vi "Begin.vi"(8 "error in":errorcluster) -> (0 "error out":errorcluster)   [LabVIEW 2014]
doc: "Called before other user functions, this VI is expected to open initial I/O refnums, load in file data, and do all program initialization. Notice that the <B>error out</B> terminal is simply used for data flow. Wiring it to other structures or subVIs ensures that this VI runs first."
uses:
  <vilib>/Rock Robotics/WPI/DriverStation/WPI_DriverStationRobotMode2.ctl
  <vilib>/Rock Robotics/WPI/Joystick/WPI_JoystickDeviceEnum.ctl
  <vilib>/Rock Robotics/WPI/CAN/TalonSRX/WPI_CANTalonSRX_APIControlMode.ctl
  <vilib>/Rock Robotics/WPI/RobotDrive/WPI_RobotDriveMotorSelectorEnum.ctl
  <vilib>/Rock Robotics/SystemInterfaces/Typedef/FPGA_TypedefDigitalModule.ctl
  Robot Global Data.vi
  <vilib>/Rock Robotics/WPI/Compressor/WPI_CompressorGetSetRefNum.vi
  <vilib>/Rock Robotics/WPI/MotorControl/WPI_MotorControlOpenCANTalonSRX.vi
  <vilib>/Rock Robotics/WPI/Solenoid/WPI_SolenoidOpenSingle.vi
  <vilib>/Rock Robotics/WPI/Solenoid/WPI_SolenoidOpenDouble.vi
  <vilib>/Rock Robotics/WPI/Switch/WPI_SwitchOpenLimit.vi
  <vilib>/Rock Robotics/WPI/RobotDrive/WPI_RobotDriveOpen4MotorWithExistingMotors.vi
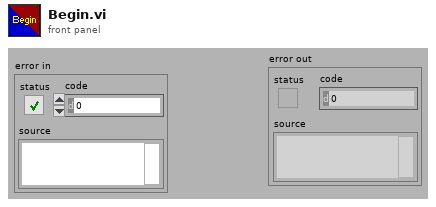
[diagram p1: front panel]
types:
  T1 = typedef "FPGA_TypedefDigitalModule.ctl" = enum16{"Controller 1"}
  T2 = typedef "WPI_JoystickDeviceEnum.ctl" = enum16{"USB 0", "USB 1", "USB 2", "USB 3", "USB 4", "USB 5"}
  T3 = typedef "WPI_RobotDriveMotorSelectorEnum.ctl" = enum16{"Rear Left Motor", "Rear Right Motor", "Front Left Motor", "Front Right Motor"}
  T4 = typedef "WPI_CANTalonSRX_APIControlMode.ctl" = enum8{"Percent VBus", "Speed", "Position", "Slave", "Unchanged / Invalid"}
  T5 = typedef "WPI_DriverStationRobotMode2.ctl" = enum16{"Autonomous Disabled", "Autonomous Enabled", "Teleop Disabled", "Teleop Enabled", "Disconnected", "Finish", "Test Disabled", "Test Enabled", "Emergency Stopped"}
  T6 = typedef "WPI_MotorControlDeviceRef.ctl" = cluster{"DeviceStatus":errorcluster, "Type":T7, "PWM":cluster{"Controller":T1, "PWM Channel":T8, "DeadBand":T9}, "CAN":cluster{"Device Number":u8, "Control Mode":T10, "Semaphore":T11, "Max Vout":dbl, "TalonSRX Control Mode":T4}, "Invert":bool, "TransformRef":T12, "InvTransformRef":T12}
  T7 = typedef "WPI_MotorControlType.ctl" = enum16{"PWM", "CAN", "CANTalonSRX"}
  T8 = typedef "FPGA_DIOPWMChannel.ctl" = enum8{"PWM 0", "PWM 1", "PWM 2", "PWM 3", "PWM 4", "PWM 5", "PWM 6", "PWM 7", "PWM 8", "PWM 9", "PWM MXP 0", "PWM MXP 1", "PWM MXP 2", "PWM MXP 3", "PWM MXP 4", "PWM MXP 5", "PWM MXP 6", "PWM MXP 7", "PWM MXP 8", "PWM MXP 9", "Invalid"}
  T9 = typedef "WPI_PWMDeadband.ctl" = cluster{"Name":string, "maxPositivePwm":i32, "minPositivePwm":i32, "centerPwm":i32, "maxNegativePwm":i32, "minNegativePwm":i32, "angularRange":u16}
  T10 = typedef "WPI_CANJaguar_ControlMode.ctl" = enum8{"Percent VBus", "Current", "Speed", "Position", "Voltage"}
  T11 = typedef "Semaphore RefNum" = refnum<k1>
  T12 = typedef "WPI_PWMTransform_ConPane.ctl" = refnum<vi>
  T13 = typedef "WPI_SolenoidDevRef.ctl" = cluster{"DevStatus":errorcluster, "Pneumatics Control Module":u8, "Forward Solenoid Channel":T14, "Reverse Solenoid Channel":T14}
  T14 = typedef "WPI_SolenoidChannel.ctl" = enum8{"Solenoid 0", "Solenoid 1", "Solenoid 2", "Solenoid 3", "Solenoid 4", "Solenoid 5", "Solenoid 6", "Solenoid 7", "Invalid"}
  T15 = typedef "WPI_RobotDriveDevRef.ctl" = cluster{"DevStatus":errorcluster, "Motors[]":T6[], "Square Inputs":bool, "Max Output":dbl}
  T16 = typedef "WPI_JoystickDevRef.ctl" = cluster{"Device":T2}
  T17 = typedef "FPGA_DIOChannel.ctl" = enum8{"DIO 0", "DIO 1", "DIO 2", "DIO 3", "DIO 4", "DIO 5", "DIO 6", "DIO 7", "DIO 8", "DIO 9", "DIO MXP 0", "DIO MXP 1", "DIO MXP 2", "DIO MXP 3", "DIO MXP 4", "DIO MXP 5", "DIO MXP 6", "DIO MXP 7", "DIO MXP 8", "DIO MXP 9", "DIO MXP 10", "DIO MXP 11", "DIO MXP 12", "DIO MXP 13", "DIO MXP 14", "DIO MXP 15", "Invalid"}
  T18 = typedef "WPI_CompressorDevRef.ctl" = cluster{"DevStatus":errorcluster, "Pneumatics Control Module":u8}
  T19 = typedef "WPI_SwitchDevRef.ctl" = cluster{"DevStatus":errorcluster, "DIO Channel":T17, "Controller":T1, "CntIndex":T20, "Normally Closed":bool}
  T20 = typedef "FPGA_CounterCtrSystemIndex.ctl" = enum8{"Ctr 0", "Ctr 1", "Ctr 2", "Ctr 3", "Ctr 4", "Ctr 5", "Ctr 6", "Ctr 7", "Invalid"}
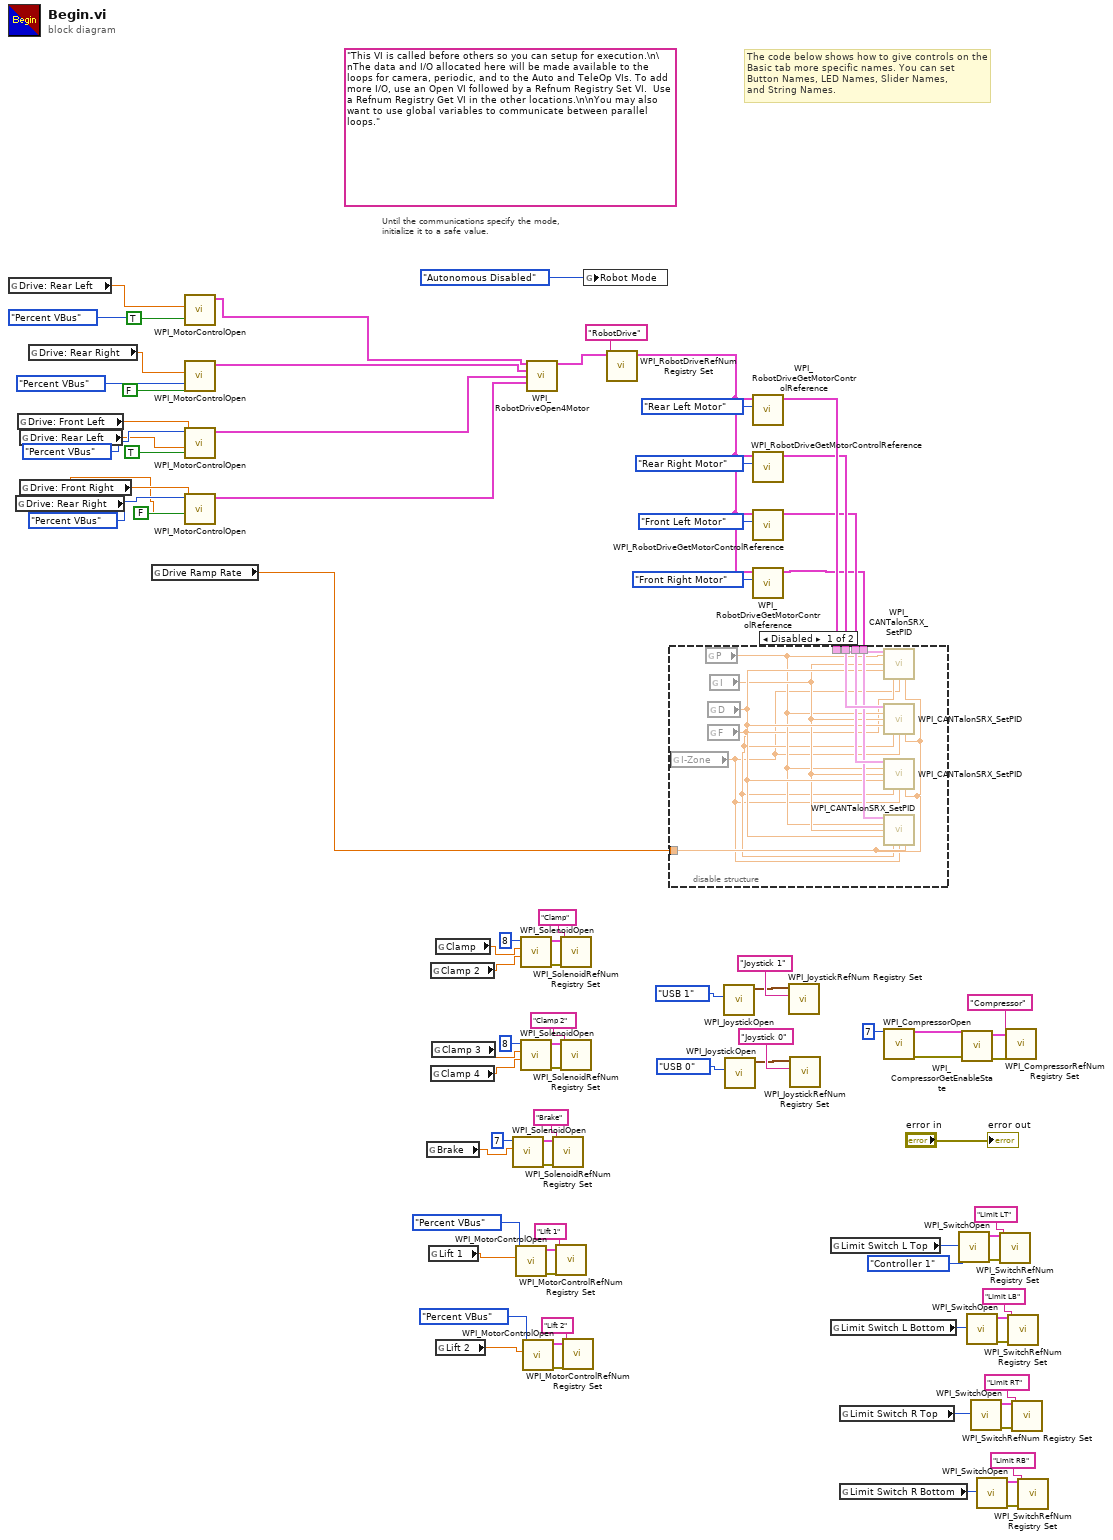
[diagram p0: block diagram]
diagram:
  (unwired) "This VI is called before others so you can setup for execution.\n\nThe data and I/O allocated here will be made available to the loops for camera, periodic, and to the Auto and TeleOp VIs. To add more I/O, use an Open VI followed by a Refnum Registry Set VI.  Use a Refnum Registry Get VI in the other locations.\n\nYou may also want to use global variables to communicate between parallel loops."
  # "The code below shows how to give controls on the\nBasic tab more specific names. You can set\nButton Names, LED Names, Slider Names,\nand String Names."
  # "Until the communications specify the mode,\ninitialize it to a safe value."
  n1 = global read "Robot Global Data.vi" "Drive: Rear Left"() -> (w80:dbl)
  n2 = global read "Robot Global Data.vi" "Drive: Rear Right"() -> (w2:dbl)
  n3 = global read "Robot Global Data.vi" "Drive: Front Left"() -> (w81:dbl)
  n4 = global read "Robot Global Data.vi" "Drive: Rear Left"() -> (w1:dbl)
  n5 = global read "Robot Global Data.vi" "Drive: Front Right"() -> (w82:dbl)
  n6 = global read "Robot Global Data.vi" "Drive: Rear Right"() -> (w83:dbl)
  n7 = global read "Robot Global Data.vi" "Drive Ramp Rate"() -> (w42:dbl)
  n8 = call-poly <vilib>:"WPI_MotorControlOpen.vi"("Invert"=TRUE, "Device Number"=w80, "Control Mode"=WPI_CANTalonSRX_APIControlMode."Percent VBus") -> ("MotorControlDeviceRef"=w53:T6)  [unwired: 7 in, 1 out]
  n9 = call-poly <vilib>:"WPI_MotorControlOpen.vi"("Invert"=FALSE, "Device Number"=w83, "Control Mode"=WPI_CANTalonSRX_APIControlMode."Percent VBus") -> ("MotorControlDeviceRef"=w52:T6)  [unwired: 7 in, 1 out]
  n10 = call-poly <vilib>:"WPI_MotorControlOpen.vi"("Invert"=TRUE, "Master Device Number"=w1, "Device Number"=w81, "Control Mode"=WPI_CANTalonSRX_APIControlMode."Percent VBus") -> ("MotorControlDeviceRef"=w51:T6)  [unwired: 6 in, 1 out]
  n11 = call-poly <vilib>:"WPI_MotorControlOpen.vi"("Invert"=FALSE, "Master Device Number"=w2, "Device Number"=w82, "Control Mode"=WPI_CANTalonSRX_APIControlMode."Percent VBus") -> ("MotorControlDeviceRef"=w37:T6)  [unwired: 6 in, 1 out]
  n12 = global read "Robot Global Data.vi" "Brake"() -> (w71:dbl)
  n13 = global read "Robot Global Data.vi" "Lift 1"() -> (w63:dbl)
  n14 = global read "Robot Global Data.vi" "Clamp 2"() -> (w8:dbl)
  n15 = global read "Robot Global Data.vi" "Clamp 4"() -> (w55:dbl)
  n16 = global read "Robot Global Data.vi" "Clamp 3"() -> (w60:dbl)
  n17 = global read "Robot Global Data.vi" "Clamp"() -> (w13:dbl)
  n18 = global read "Robot Global Data.vi" "Lift 2"() -> (w15:dbl)
  n19 = call-poly <vilib>:"WPI_SolenoidOpen.vi"("Solenoid Channel"=w71, "Pneumatics Control Module (0)"=u8 7) -> ("error out"=w70:errorcluster, "SolenoidDevRef"=w69:T13)  [unwired: 8 in]
  n20 = call-poly <vilib>:"WPI_MotorControlOpen.vi"("Device Number"=w63, "Control Mode"=WPI_CANTalonSRX_APIControlMode."Percent VBus") -> ("error out"=w67:errorcluster, "MotorControlDeviceRef"=w49:T6)  [unwired: 8 in]
  n21 = call-poly <vilib>:"WPI_SolenoidOpen.vi"("Reverse Solenoid Channel"=w8, "Forward Solenoid Channel"=w13, "Pneumatics Control Module (0)"=u8 8) -> ("error out"=w12:errorcluster, "SolenoidDevRef"=w11:T13)  [unwired: 7 in]
  n22 = call-poly <vilib>:"WPI_SolenoidOpen.vi"("Reverse Solenoid Channel"=w55, "Forward Solenoid Channel"=w60, "Pneumatics Control Module (0)"=u8 8) -> ("error out"=w59:errorcluster, "SolenoidDevRef"=w58:T13)  [unwired: 7 in]
  n23 = call-poly <vilib>:"WPI_MotorControlOpen.vi"("Device Number"=w15, "Control Mode"=WPI_CANTalonSRX_APIControlMode."Percent VBus") -> ("error out"=w61:errorcluster, "MotorControlDeviceRef"=w48:T6)  [unwired: 8 in]
  n24 = call-poly <vilib>:"WPI_RobotDriveOpen4Motor.vi"("Rear Left Motor Dev Ref"=w53, "Rear Right Motor Dev Ref"=w52, "Front Left Motor Dev Ref"=w51, "Front Right Motor Dev Ref"=w37) -> ("RobotDriveDevRef"=w54:T15)  [unwired: 10 in, 1 out]
  n25 = call <vilib>:"WPI_SolenoidRefNum Registry Set.vi"("error in (no error)"=w70, "refnum name"="Brake", "SolenoidDevRef"=w69) -> ()  [unwired: 7 in, 2 out]
  n26 = call <vilib>:"WPI_MotorControlRefNum Registry Set.vi"("error in (no error)"=w67, "refnum name"="Lift 1", "MotorControlDevRef"=w49) -> ()  [unwired: 7 in, 2 out]
  n27 = call <vilib>:"WPI_SolenoidRefNum Registry Set.vi"("error in (no error)"=w12, "refnum name"="Clamp", "SolenoidDevRef"=w11) -> ()  [unwired: 7 in, 2 out]
  n28 = call <vilib>:"WPI_SolenoidRefNum Registry Set.vi"("error in (no error)"=w59, "refnum name"="Clamp 2", "SolenoidDevRef"=w58) -> ()  [unwired: 7 in, 2 out]
  n29 = call <vilib>:"WPI_MotorControlRefNum Registry Set.vi"("error in (no error)"=w61, "refnum name"="Lift 2", "MotorControlDevRef"=w48) -> ()  [unwired: 7 in, 2 out]
  n30 = global write "Robot Global Data.vi" "Robot Mode"(WPI_DriverStationRobotMode2."Autonomous Disabled" ("Robot Mode")) -> ()
  n31 = call <vilib>:"WPI_RobotDriveRefNum Registry Set.vi"("refnum name"="RobotDrive", "RobotDriveDevRef"=w54) -> ("RobotDriveDevRef"=w43:T15)  [unwired: 1 in, 8 out]
  n32 = call <vilib>:"WPI_JoystickOpen.vi"("JoystickDevice"=WPI_JoystickDeviceEnum."USB 1") -> ("JoystickDevRef"=w40:T16)  [unwired: 10 in]
  n33 = call <vilib>:"WPI_JoystickOpen.vi"("JoystickDevice"=WPI_JoystickDeviceEnum."USB 0") -> ("JoystickDevRef"=w86:T16)  [unwired: 10 in]
  n34 = call <vilib>:"WPI_RobotDriveGetMotorControlReference.vi"("MotorIndex"=WPI_RobotDriveMotorSelectorEnum."Rear Left Motor", "RobotDriveDevRef"=w43) -> ("MotorControlDeviceRef"=w36:T6)  [unwired: 9 out]
  n35 = call <vilib>:"WPI_RobotDriveGetMotorControlReference.vi"("MotorIndex"=WPI_RobotDriveMotorSelectorEnum."Rear Right Motor", "RobotDriveDevRef"=w43) -> ("MotorControlDeviceRef"=w35:T6)  [unwired: 9 out]
  n36 = call <vilib>:"WPI_RobotDriveGetMotorControlReference.vi"("MotorIndex"=WPI_RobotDriveMotorSelectorEnum."Front Left Motor", "RobotDriveDevRef"=w43) -> ("MotorControlDeviceRef"=w34:T6)  [unwired: 9 out]
  n37 = call <vilib>:"WPI_RobotDriveGetMotorControlReference.vi"("MotorIndex"=WPI_RobotDriveMotorSelectorEnum."Front Right Motor", "RobotDriveDevRef"=w43) -> ("MotorControlDeviceRef"=w33:T6)  [unwired: 9 out]
  n38 = disable-structure shown="Disabled" {
    disable-tunnel: w36 -> [w98 _]
    disable-tunnel: w35 -> [w97 _]
    disable-tunnel: w34 -> [w96 _]
    disable-tunnel: w33 -> [w95 _]
    disable-tunnel: w42 -> [w91 _]
    frame Disabled {
      n39 = global read "Robot Global Data.vi" "I-Zone"() -> (w89:dbl)
      n40 = global read "Robot Global Data.vi" "P"() -> (w92:dbl)
      n41 = global read "Robot Global Data.vi" "D"() -> (w94:dbl)
      n42 = global read "Robot Global Data.vi" "F"() -> (w90:dbl)
      n43 = global read "Robot Global Data.vi" "I"() -> (w93:dbl)
      n44 = call <vilib>:"WPI_CANTalonSRX_SetPID.vi"("CAN Talon SRX Ref"=w98, "P"=w92, "I"=w93, "D"=w94, "F"=w90, "I Zone"=w89, "Ramp Rate"=w91) -> ()  [unwired: 7 in, 2 out]
      n45 = call <vilib>:"WPI_CANTalonSRX_SetPID.vi"("CAN Talon SRX Ref"=w97, "P"=w92, "I"=w93, "D"=w94, "F"=w90, "I Zone"=w89, "Ramp Rate"=w91) -> ()  [unwired: 7 in, 2 out]
      n46 = call <vilib>:"WPI_CANTalonSRX_SetPID.vi"("CAN Talon SRX Ref"=w96, "P"=w92, "I"=w93, "D"=w94, "F"=w90, "I Zone"=w89, "Ramp Rate"=w91) -> ()  [unwired: 7 in, 2 out]
      n47 = call <vilib>:"WPI_CANTalonSRX_SetPID.vi"("CAN Talon SRX Ref"=w95, "P"=w92, "I"=w93, "D"=w94, "F"=w90, "I Zone"=w89, "Ramp Rate"=w91) -> ()  [unwired: 7 in, 2 out]
    }
    frame Enabled {
    }
  }
  n48 = call <vilib>:"WPI_JoystickRefNum Registry Set.vi"("refnum name"="Joystick 1", "JoystickDevRef"=w40) -> ()  [unwired: 8 in, 2 out]
  n49 = call <vilib>:"WPI_JoystickRefNum Registry Set.vi"("refnum name"="Joystick 0", "JoystickDevRef"=w86) -> ()  [unwired: 8 in, 2 out]
  n50 = global read "Robot Global Data.vi" "Limit Switch L Top"() -> (w31:T17)
  n51 = global read "Robot Global Data.vi" "Limit Switch L Bottom"() -> (w27:T17)
  n52 = global read "Robot Global Data.vi" "Limit Switch R Top"() -> (w20:T17)
  n53 = global read "Robot Global Data.vi" "Limit Switch R Bottom"() -> (w19:T17)
  n54 = call <vilib>:"WPI_CompressorOpen.vi"("Pneumatics Control Module (0)"=u8 7) -> ("CompressorDevRef"=w7:T18, "error out"=w6:errorcluster)  [unwired: 13 in]
  n55 = call-poly <vilib>:"WPI_SwitchOpen.vi"("DIO Channel"=w31, "Controller"=FPGA_TypedefDigitalModule."Controller 1") -> ("error out"=w30:errorcluster, "SwitchDevRef"=w29:T19)  [unwired: 8 in]
  n56 = call <vilib>:"WPI_CompressorGetEnableState.vi"("error in (no error)"=w6, "CompressorDevRef"=w7) -> ("error out"=w5:errorcluster, "CompressorDevRef"=w4:T18)  [unwired: 6 in, 2 out]
  n57 = call-poly <vilib>:"WPI_SwitchOpen.vi"("DIO Channel"=w27) -> ("error out"=w26:errorcluster, "SwitchDevRef"=w25:T19)  [unwired: 9 in]
  n58 = call-poly <vilib>:"WPI_SwitchOpen.vi"("DIO Channel"=w20) -> ("error out"=w21:errorcluster, "SwitchDevRef"=w22:T19)  [unwired: 9 in]
  n59 = call-poly <vilib>:"WPI_SwitchOpen.vi"("DIO Channel"=w19) -> ("error out"=w18:errorcluster, "SwitchDevRef"=w17:T19)  [unwired: 9 in]
  n60 = call <vilib>:"WPI_SwitchRefNum Registry Set.vi"("error in (no error)"=w30, "refnum name"="Limit LT", "SwitchDevRef"=w29) -> ()  [unwired: 7 in, 2 out]
  n61 = call <vilib>:"WPI_CompressorRefNum Registry Set.vi"("error in (no error)"=w5, "refnum name"="Compressor", "CompressorDevRef"=w4) -> ()  [unwired: 7 in, 2 out]
  n62 = call <vilib>:"WPI_SwitchRefNum Registry Set.vi"("error in (no error)"=w26, "refnum name"="Limit LB", "SwitchDevRef"=w25) -> ()  [unwired: 7 in, 2 out]
  n63 = call <vilib>:"WPI_SwitchRefNum Registry Set.vi"("error in (no error)"=w21, "refnum name"="Limit RT", "SwitchDevRef"=w22) -> ()  [unwired: 7 in, 2 out]
  n64 = call <vilib>:"WPI_SwitchRefNum Registry Set.vi"("error in (no error)"=w18, "refnum name"="Limit RB", "SwitchDevRef"=w17) -> ()  [unwired: 7 in, 2 out]
  "error out" <- "error in"
